vi "WPI_DigitalModuleGetDIO.vi"(8 "error in (no error)":errorcluster, 10 "DIOChannel":T1=enum."DIO 1", 11 "DigitalModuleDevRef":T2) -> (0 "error out":errorcluster, 2 "Value":bool, 3 "DigitalModuleDevRef":T2)   [LabVIEW 2017]
doc: "This software is licensed. Open the labview\\readme\\WPI Robotics Library Open Source License.txt file for more information."
uses:
  <vilib>/Rock Robotics/WPI/DigitalModule/WPI_DigitalModuleDeviceRef.ctl
  <vilib>/Rock Robotics/SystemInterfaces/DIO/FPGA_DIOChannel.ctl
  <vilib>/Rock Robotics/SystemInterfaces/System/FPGA_SystemGet.vi
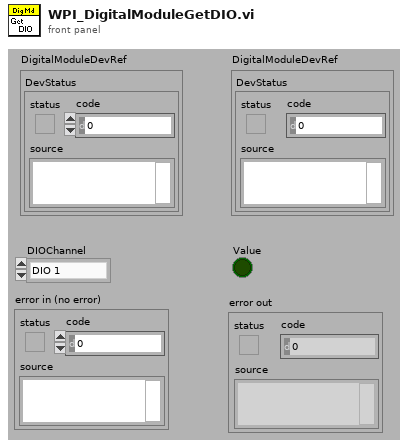
[diagram p1: front panel]
types:
  T1 = typedef "FPGA_DIOChannel.ctl" = enum8{"DIO 0", "DIO 1", "DIO 2", "DIO 3", "DIO 4", "DIO 5", "DIO 6", "DIO 7", "DIO 8", "DIO 9", "DIO MXP 0", "DIO MXP 1", "DIO MXP 2", "DIO MXP 3", "DIO MXP 4", "DIO MXP 5", "DIO MXP 6", "DIO MXP 7", "DIO MXP 8", "DIO MXP 9", "DIO MXP 10", "DIO MXP 11", "DIO MXP 12", "DIO MXP 13", "DIO MXP 14", "DIO MXP 15", "SPI Port CS1", "SPI Port CS2", "SPI Port CS3", "SPI Port MISO", "SPI Port MOSI", "Invalid"}
  T2 = typedef "WPI_DigitalModuleDeviceRef.ctl" = cluster{"DevStatus":errorcluster}
  T3 = typedef "FPGA_DIODevRef.ctl" = cluster{"DevStatus":errorcluster}
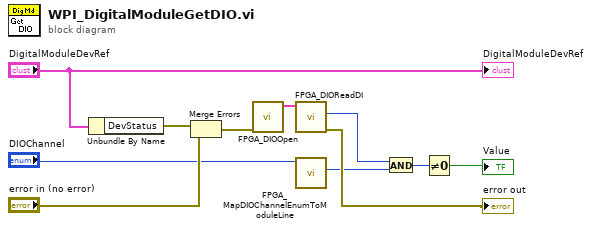
[diagram p0: block diagram]
diagram:
  n1 = Unbundle By Name("DigitalModuleDevRef") -> ("DevStatus"=w3:errorcluster)
  n2 = Merge Errors(w3, "error in (no error)") -> (w2:errorcluster)
  n3 = call <vilib>:"FPGA_DIOOpen.vi"("error in (no error)"=w2) -> ("DIODeviceRef"=w6:T3)  [unwired: 1 in, 9 out]
  n4 = call <vilib>:"FPGA_DIOReadDI.vi"("DIODeviceRef"=w6) -> ("error out"=→"error out":errorcluster, "DI"=w5:u32)  [unwired: 1 in, 8 out]
  n5 = call <vilib>:"FPGA_MapDIOChannelEnumToModuleLine.vi"("DIOChannel"="DIOChannel") -> ("ActualDIOBitMask(U32)"=w4:u32)  [unwired: 10 out]
  n6 = And(x=w5, y=w4) -> (x .and. y?=w7:u32)
  n7 = Not Equal To 0?(x=w7) -> (x != 0?=→"Value":bool)
  "DigitalModuleDevRef" <- "DigitalModuleDevRef"
